vi "Get System Configuration.vi"(4 "error in (no error)":errorcluster, 7 "VISA resource name":refnum<visa-resource-name>) -> (0 "error out":errorcluster, 2 "System Configuration":T1, 3 "VISA resource name out":refnum<visa-resource-name>)   [LabVIEW 2012, in "Newport ESP301.lvlib"]
doc: "Get system fault checking, event handling and general setup for all axes."
uses:
  Newport ESP301.lvlib
panel:
  # "queue purge on time expiration disabled"
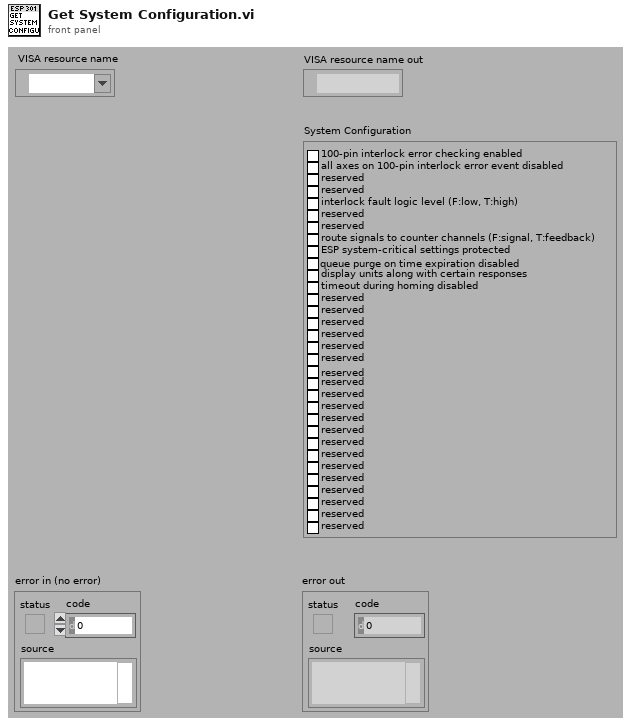
[diagram p1: front panel]
types:
  T1 = cluster{"100-pin interlock error checking enabled":bool, "all axes on 100-pin interlock error event disabled":bool, "reserved":bool, "reserved":bool, "interlock fault logic level (F:low, T:high)":bool, "reserved":bool, "reserved":bool, "route signals to counter channels (F:signal, T:feedback)":bool, "ESP system-critical settings protected":bool, bool, "display units along with certain responses ":bool, "timeout during homing disabled ":bool, "reserved ":bool, "reserved ":bool, "reserved ":bool, "reserved ":bool, "reserved ":bool, "reserved ":bool, "reserved ":bool, "reserved ":bool, "reserved ":bool, "reserved ":bool, "reserved ":bool, "reserved ":bool, "reserved ":bool, "reserved ":bool, "reserved ":bool, "reserved ":bool, "reserved ":bool, "reserved ":bool, "reserved ":bool, "reserved":bool}
  T2 = cluster{"Boolean array[0]":bool, "Boolean array[1]":bool, "Boolean array[2]":bool, "Boolean array[3]":bool, "Boolean array[4]":bool, "Boolean array[5]":bool, "Boolean array[6]":bool, "Boolean array[7]":bool, "Boolean array[8]":bool, "Boolean array[9]":bool, "Boolean array[10]":bool, "Boolean array[11]":bool, "Boolean array[12]":bool, "Boolean array[13]":bool, "Boolean array[14]":bool, "Boolean array[15]":bool, "Boolean array[16]":bool, "Boolean array[17]":bool, "Boolean array[18]":bool, "Boolean array[19]":bool, "Boolean array[20]":bool, "Boolean array[21]":bool, "Boolean array[22]":bool, "Boolean array[23]":bool, "Boolean array[24]":bool, "Boolean array[25]":bool, "Boolean array[26]":bool, "Boolean array[27]":bool, "Boolean array[28]":bool, "Boolean array[29]":bool, "Boolean array[30]":bool, "Boolean array[31]":bool}
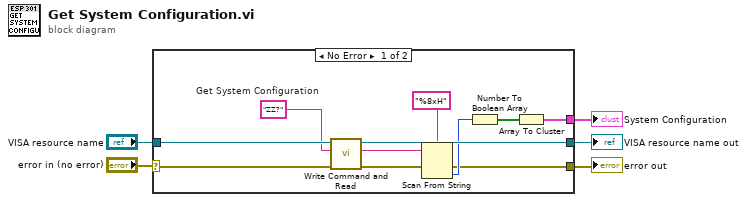
[diagram p0: block diagram]
diagram:
  n1 = case shown="No Error" "error in (no error)" {
    selector: "error in (no error)" -> [w14 w18]
    tunnel: [w8 w18] -> w5
    tunnel: "VISA resource name" -> [w16 w17]
    tunnel: [w15 w17] -> w4
    tunnel: [w7 _] -> w1
    frame No Error {
      w13 = "ZZ?"  # Get System Configuration
      n2 = call "Write Command and Read.vi"("error in (no error)"=w14, "Command"=w13, "VISA resource name"=w16) -> ("error out"=w9:errorcluster, "Returned string"=w6:string, "VISA resource name out"=w15:refnum<visa-resource-name>)  [unwired: 2 in, 2 out]
      n3 = Scan From String(format string="%8xH" ("chaîne de format"), input string=w6, error in=w9) -> (error out=w8:errorcluster, output 1=w10:u32)  [unwired: 2 in, 2 out]
      n4 = Number To Boolean Array(number=w10) -> (Boolean array=w12:bool[])
      n5 = Array To Cluster(array=w12) -> (cluster=w7:T2)
    }
    frame Error {
    }
  }
  "error out" <- w5
  "VISA resource name out" <- w4
  "System Configuration" <- w1
